vi "Get_Sweep_Speed_table.vi"(8 "error in (no error)":errorcluster, 11 ".NET Reference in":refnum<k24>) -> (0 "error out":errorcluster, 2 "Get_Sweep_Speed_table":dbl[](array[numeric]), 3 "Reference out":refnum<k24>)   [LabVIEW 2017]
uses:
  C:/Users/Ssantec_Test/Documents/Instrument_DLL_Sample_Labview_20220902_Ver1.2.2/DLL/x86/InstrumentDLL.dll
  DLL/x86/InstrumentDLL.dll
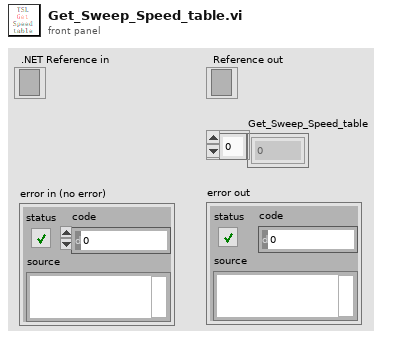
[diagram p1: front panel]
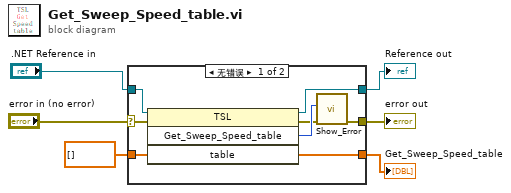
[diagram p0: block diagram]
diagram:
  n1 = case shown="无错误" "error in (no error)" {
    selector: "error in (no error)" -> [w9 w17]
    tunnel: [w14 w15] -> w6
    tunnel: [w10 w17] -> w5
    tunnel: dbl[] [] ("table") -> [w13 w15]
    tunnel: ".NET Reference in" -> [w8 w16]
    tunnel: [w7 w16] -> w1
    frame No Error {
      n2 = invoke on="调用节点" class="TSL" method="Get_Sweep_Speed_table"(reference=w8, error in=w9, "table"=w13) -> (reference out=w7:refnum<k24>, error out=w11:errorcluster, "Get_Sweep_Speed_table"=w12:i32, "table"=w14:dbl[])  [unwired: 1 in]
      n3 = call "Show_Error.vi"("error in (no error)"=w11, "Error"=w12) -> ("error out"=w10:errorcluster)  [unwired: 9 in]
    }
    frame Error {
    }
  }
  "Get_Sweep_Speed_table" <- w6
  "error out" <- w5
  "Reference out" <- w1
